vi "Scope Tester.vi"() -> ()   [LabVIEW 2018]
uses:
  src/api/logger_class/Failure Information.ctl
  src/api/logger_class/Log Record.ctl
  src/api/logger_class/Internal Log Levels.ctl
  src/api/logger_class/Log Levels.ctl
  src/api/configuration/scopes/basic_scope/Basic.lvclass
  C:/Users/Colin/Documents/software_projects/labview/glog/src/api/extension/scope_interface/Scope.lvclass
  src/api/configuration/scopes/basic_scope/New (Element).vi
  src/api/logger_class/Log (Parts).vi
  src/api/logger_class/Logger.lvclass
  Scope Tester Class.lvclass
  Scope Tester Library.lvlib
panel:
  out "failure info":T1 {"Log Record"."timestamp" format="%<%x %.3X>T"}
  out "error out":errorcluster
  # "Locals"
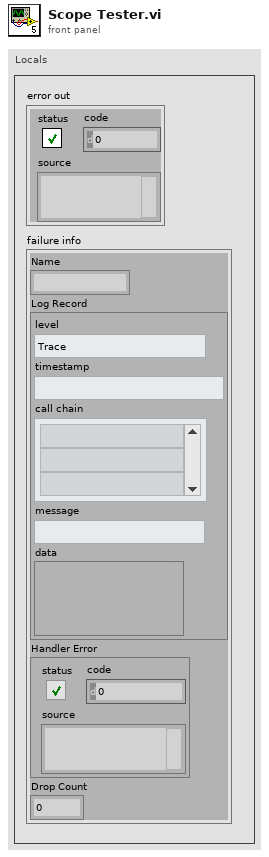
[diagram p1: front panel]
types:
  T1 = typedef "GLog.lvlib/Logger.lvclass/Failure Information.ctl" = cluster{"Name":string, "Log Record":T2, "Handler Error":errorcluster, "Drop Count":u32}
  T2 = typedef "GLog.lvlib/Logger.lvclass/Log Record.ctl" = cluster{"level":T3, "timestamp":timestamp, "call chain":string[], "message":string, "data":variant}
  T3 = typedef "GLog.lvlib/Logger.lvclass/Internal Log Levels.ctl" = enum16{"Trace", "Debug", "Info", "Warning", "Error", "Critical", "Internal"}
  T4 = typedef "GLog.lvlib/Logger.lvclass/Log Levels.ctl" = enum16{"Trace", "Debug", "Info", "Warning", "Error", "Critical"}
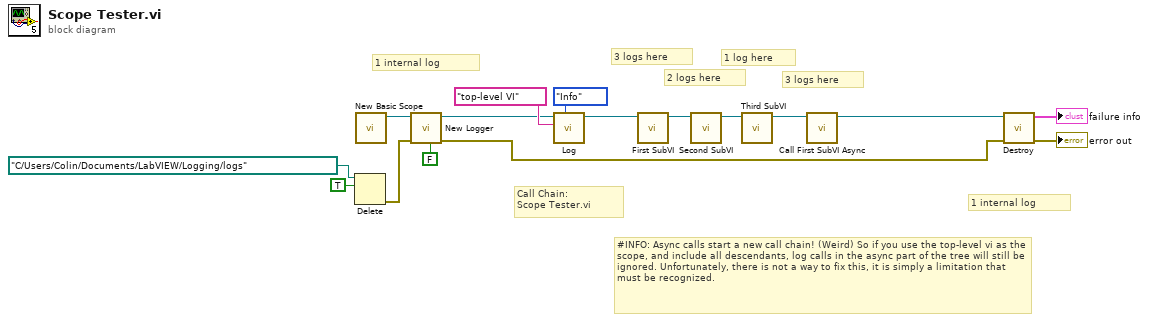
[diagram p0: block diagram]
diagram:
  # "#INFO: Async calls start a new call chain! (Weird) So if you use the top-level vi as the scope, and include all descendants, log calls in the async part of the tree will still be ignored. Unfortunately, there is not a way to fix this, it is simply a limitation that must be recognized."
  # "3 logs here"
  # "1 log here"
  # "2 logs here"
  # "1 internal log"
  # "3 logs here"
  # "Call Chain:\nScope Tester.vi"
  # "1 internal log"
  n1 = Delete(path (use dialog)=path "C:/Users/Colin/Documents/LabVIEW/Logging/logs", entire hierarchy (F)=TRUE) -> (error out=w5:errorcluster)  [unwired: 3 in, 2 out]
  n2 = call-poly "New Basic Scope.vi"() -> ("basic scope"=w16:refnum<class "Basic.lvclass">)  [unwired: 11 in]
  n3 = call "New Logger.vi"("dialog on failure? (T)"=FALSE, "error in (no error)"=w5, "logger scope (all)"=w16) -> ("error out"=w10:errorcluster, "logger"=w14:refnum<class "Logger.lvclass">)  [unwired: 7 in]
  n4 = call-poly "Log.vi"("log level"=Log_Levels."Info" ("level"), "message"="top-level VI", "logger in"=w14) -> ("logger out"=w12:refnum<class "Logger.lvclass">)  [unwired: 8 in]
  n5 = call "First SubVI.vi"("logger in"=w12) -> ("logger out"=w4:refnum<class "Logger.lvclass">)  [unwired: 10 in]
  n6 = call "Second SubVI.vi"("logger in"=w4) -> ("logger out"=w3:refnum<class "Logger.lvclass">)  [unwired: 10 in]
  n7 = call "Third SubVI.vi"("logger in"=w3) -> ("logger out"=w2:refnum<class "Logger.lvclass">)  [unwired: 10 in]
  n8 = call "Call First SubVI Async.vi"("logger in"=w2) -> ("logger out"=w1:refnum<class "Logger.lvclass">)  [unwired: 10 in]
  n9 = call "Destroy.vi"("error in (no error)"=w10, "logger in"=w1) -> ("error out"=→"error out":errorcluster, "failure info"=→"failure info":T1)  [unwired: 8 in]
